vi "校准记录.vi"(8 "error in (no error)":errorcluster, 9 "曲线模型":T1={"标液浓度1"=0.0, "测量吸光度1"=0.0, "样品1启用"=FALSE, "标液浓度2"=0.0, "测量吸光度2"=0.0, "样品2启用"=FALSE, "标液浓度3"=0.0, "测量吸光度3"=0.0, "样品3启用"=FALSE, "标液浓度4"=0.0, "测量吸光度4"=0.0, "样品4启用"=FALSE, "标液浓度5"=0.0, "测量吸光度5"=0.0, "样品5启用"=FALSE, "模型"=enum."线性", "精度"=4.0, "XY图"=[], "拟合公式"="", "r^2"=0.0, "标样一校准时间"=timestamp(0 s since 1904-01-01), "标样二校准时间"=timestamp(0 s since 1904-01-01), "标样三校准时间"=timestamp(0 s since 1904-01-01), "标样四校准时间"=timestamp(0 s since 1904-01-01), "标样五校准时间"=timestamp(0 s since 1904-01-01), "二次方程"={"c"=0.0, "x"=0.0, "x^2"=0.0}, "标定时间"=timestamp(0 s since 1904-01-01), "拟合公式 2"="", "r^2 2"=0.0} {"r^2 2" format="%.7f"; "标定时间" format="%<%m/%d/%y %H:%M:%S>T"; "标样五校准时间" format="%<%m/%d/%y %H:%M:%S>T"; "标样四校准时间" format="%<%m/%d/%y %H:%M:%S>T"; "标样三校准时间" format="%<%m/%d/%y %H:%M:%S>T"; "标样二校准时间" format="%<%m/%d/%y %H:%M:%S>T"; "标样一校准时间" format="%<%m/%d/%y %H:%M:%S>T"; "r^2" format="%.7f"; "测量吸光度5" format="%#.6f"; "测量吸光度4" format="%#.6f"; "测量吸光度3" format="%#.6f"; "测量吸光度2" format="%#.6f"; "测量吸光度1" format="%#.6f"}, 10 "量程":enum16{"低量程", "高量程"}(ring), 11 "测量模式":string="所有测量模式") -> (0 "error out":errorcluster)   [LabVIEW 2016, in "斯坦道CODMn.lvlib"]
panel:
  out "结果字符串":string
  in  "data in":T2
  # "校准时间"
  # "标液浓度"
  # "吸光值显示"
  # "标液一"
  # "标液二"
  # "标液三"
  # "零点"
  # "跨度"
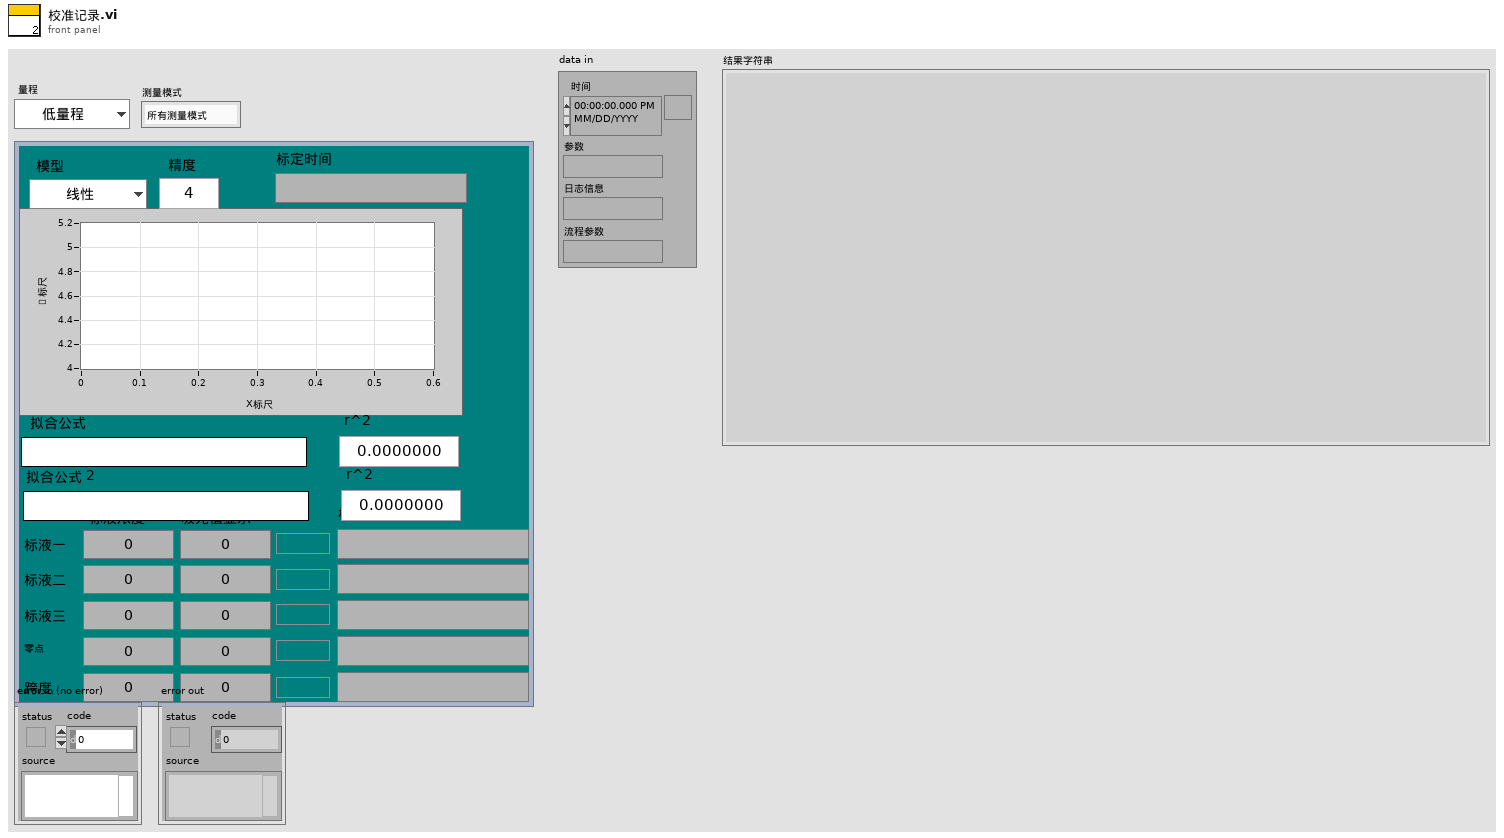
[diagram p1: front panel]
types:
  T1 = cluster{"标液浓度1":dbl, "测量吸光度1":dbl, "样品1启用":bool, "标液浓度2":dbl, "测量吸光度2":dbl, "样品2启用":bool, "标液浓度3":dbl, "测量吸光度3":dbl, "样品3启用":bool, "标液浓度4":dbl, "测量吸光度4":dbl, "样品4启用":bool, "标液浓度5":dbl, "测量吸光度5":dbl, "样品5启用":bool, "模型":enum32{"线性", "多项式", "折线"}, "精度":dbl, "XY图":cluster{"X Values":dbl[], "Y Values":dbl[]}[], "拟合公式":string, "r^2":dbl, "标样一校准时间":timestamp, "标样二校准时间":timestamp, "标样三校准时间":timestamp, "标样四校准时间":timestamp, "标样五校准时间":timestamp, "二次方程":cluster{"c":dbl, "x":dbl, "x^2":dbl}, "标定时间":timestamp, "拟合公式 2":string, "r^2 2":dbl}
  T2 = cluster{"时间":timestamp, "参数":string, "日志信息":string, "流程参数":string}
  T3 = cluster{"低标液1浓度":dbl, "低标液1信号值":dbl, "低标液1启用":u16, "低标液2浓度":dbl, "低标液2信号值":dbl, "低标液2启用":u16, "低标液3浓度":dbl, "低标液3信号值":dbl, "低标液3启用":u16, "低标液4浓度":dbl, "低标液4信号值":dbl, "低标液4启用":u16, "低标液5浓度":dbl, "低标液5信号值":dbl, "低标液5启用":u16, "高标液1浓度":dbl, "高标液1信号值":dbl, "高标液1启用":u16, "高标液2浓度":dbl, "高标液2信号值":dbl, "高标液2启用":u16, "高标液3浓度":dbl, "高标液3信号值":dbl, "高标液3启用":u16, "高标液4浓度":dbl, "高标液4信号值":dbl, "高标液4启用":u16, "高标液5浓度":dbl, "高标液5信号值":dbl, "高标液5启用":u16, "低斜率":dbl, "低截距":dbl, "低二次多项式系数":dbl, "低线性相关系数":dbl, "高斜率":dbl, "高截距":dbl, "高二次多项式系数":dbl, "高线性相关系数":dbl}
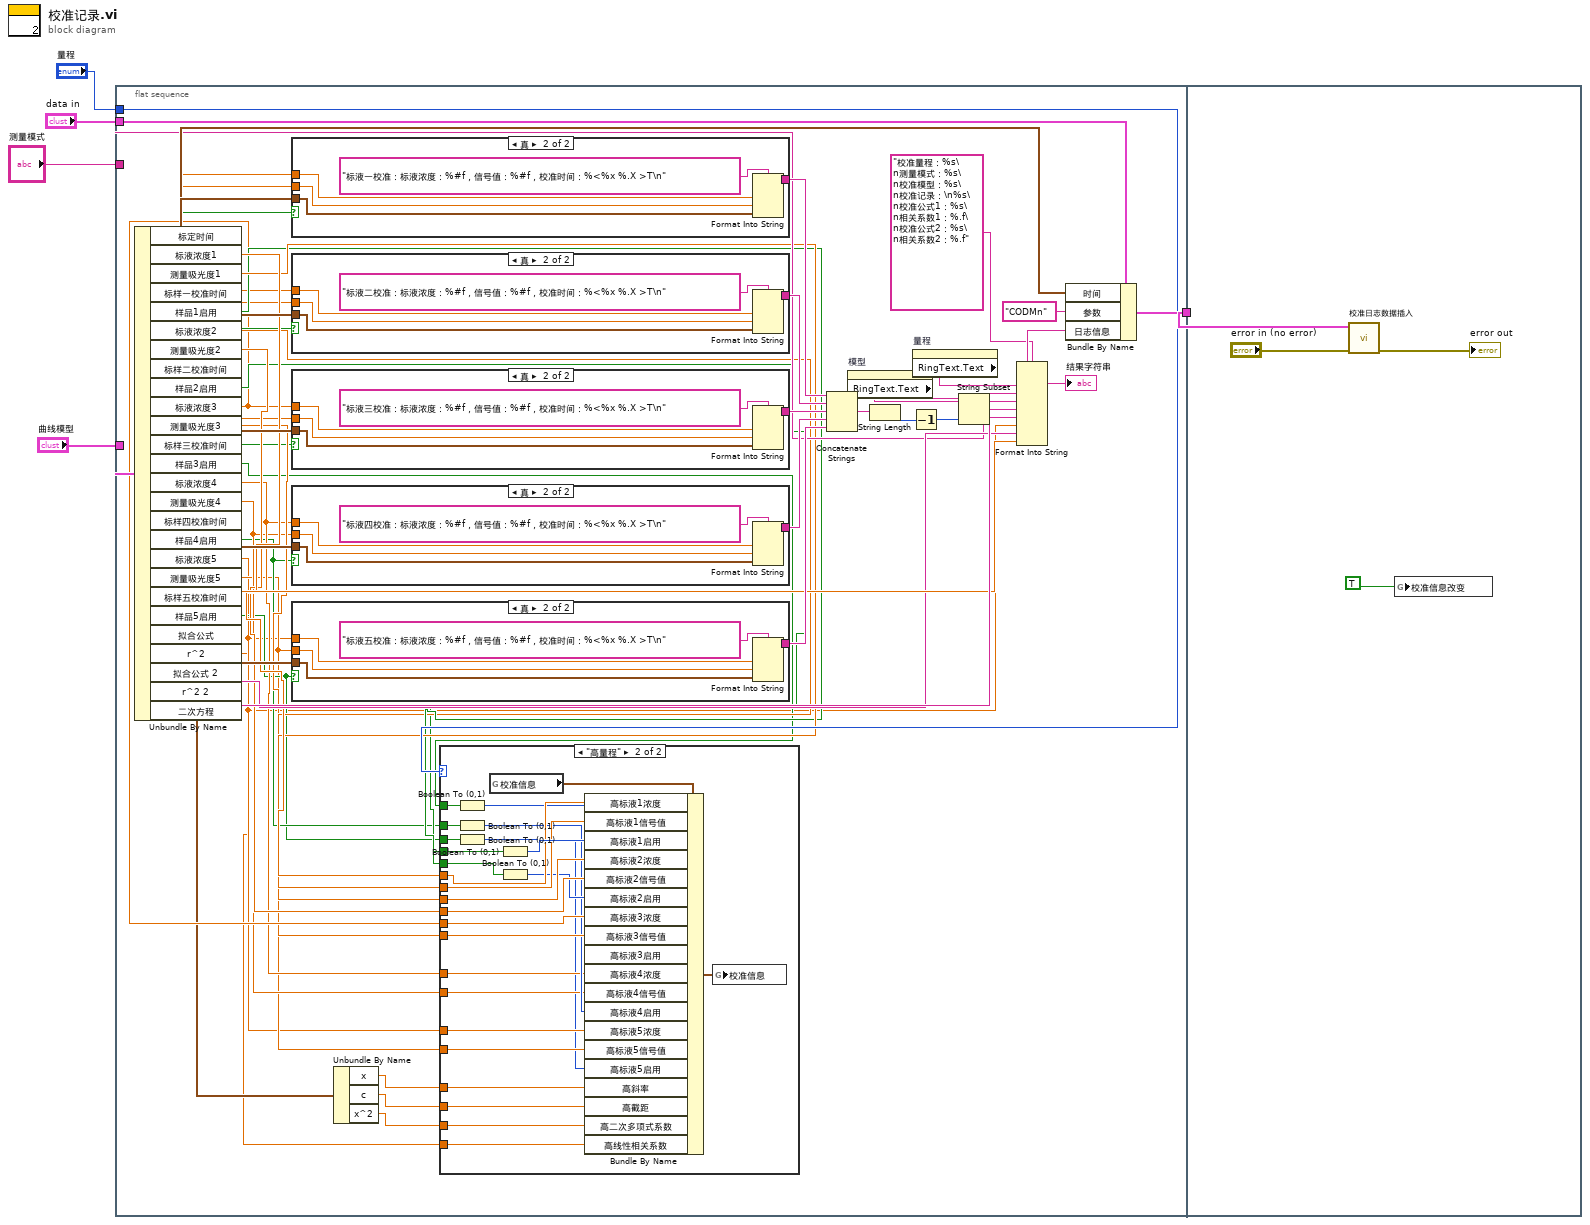
[diagram p0: block diagram]
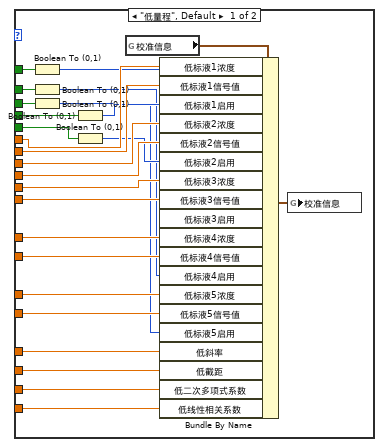
[diagram p2: hidden frame]
diagram:
  n1 = flat-sequence {
    tunnel: "量程" -> [w26]
    tunnel: "曲线模型" -> [w49]
    tunnel: "data in" -> [w53]
    tunnel: [w52] -> w2
    tunnel: "测量模式" -> [w27]
    tunnel: w2 -> [w132]
    frame #0 {
      n2 = Unbundle By Name(w49) -> ("标定时间"=w33:timestamp, "标液浓度1"=w25:dbl, "测量吸光度1"=w24:dbl, "标样一校准时间"=w48:timestamp, "样品1启用"=w23:bool, "标液浓度2"=w22:dbl, "测量吸光度2"=w21:dbl, "标样二校准时间"=w47:timestamp, "样品2启用"=w20:bool, "标液浓度3"=w19:dbl, "测量吸光度3"=w18:dbl, "标样三校准时间"=w46:timestamp, "样品3启用"=w17:bool, "标液浓度4"=w16:dbl, "测量吸光度4"=w15:dbl, "标样四校准时间"=w45:timestamp, "样品4启用"=w14:bool, "标液浓度5"=w11:dbl, "测量吸光度5"=w12:dbl, "标样五校准时间"=w44:timestamp, "样品5启用"=w13:bool, "拟合公式"=w38:string, "r^2"=w6:dbl, "拟合公式 2"=w31:string, "r^2 2"=w32:dbl, "二次方程"=w10:cluster{"c":dbl, "x":dbl, "x^2":dbl})
      n3 = case shown="真" w23 {
        tunnel: w25 -> [_ w129]
        tunnel: w24 -> [_ w128]
        tunnel: w48 -> [_ w127]
        tunnel: [_ w126] -> w43
        frame False {
        }
        frame True {
          n4 = Format Into String(format string="标液一校准：标液浓度：%#f，信号值：%#f，校准时间：%<%x %.X >T\n" ("格式字符串"), w129, w128, w127) -> (resulting string=w126:string)  [unwired: 2 in, 1 out]
        }
      }
      n5 = case shown="真" w20 {
        tunnel: w22 -> [_ w124]
        tunnel: w21 -> [_ w123]
        tunnel: w47 -> [_ w122]
        tunnel: [_ w121] -> w42
        frame False {
        }
        frame True {
          n6 = Format Into String(format string="标液二校准：标液浓度：%#f，信号值：%#f，校准时间：%<%x %.X >T\n" ("格式字符串"), w124, w123, w122) -> (resulting string=w121:string)  [unwired: 2 in, 1 out]
        }
      }
      n7 = case shown="真" w17 {
        tunnel: w19 -> [_ w119]
        tunnel: w18 -> [_ w118]
        tunnel: w46 -> [_ w117]
        tunnel: [_ w116] -> w41
        frame False {
        }
        frame True {
          n8 = Format Into String(format string="标液三校准：标液浓度：%#f，信号值：%#f，校准时间：%<%x %.X >T\n" ("格式字符串"), w119, w118, w117) -> (resulting string=w116:string)  [unwired: 2 in, 1 out]
        }
      }
      n9 = case shown="真" w14 {
        tunnel: w16 -> [_ w114]
        tunnel: w15 -> [_ w113]
        tunnel: w45 -> [_ w112]
        tunnel: [_ w111] -> w40
        frame False {
        }
        frame True {
          n10 = Format Into String(format string="标液四校准：标液浓度：%#f，信号值：%#f，校准时间：%<%x %.X >T\n" ("格式字符串"), w114, w113, w112) -> (resulting string=w111:string)  [unwired: 2 in, 1 out]
        }
      }
      n11 = case shown="真" w13 {
        tunnel: w11 -> [_ w109]
        tunnel: w12 -> [_ w108]
        tunnel: w44 -> [_ w107]
        tunnel: [_ w106] -> w39
        frame False {
        }
        frame True {
          n12 = Format Into String(format string="标液五校准：标液浓度：%#f，信号值：%#f，校准时间：%<%x %.X >T\n" ("格式字符串"), w109, w108, w107) -> (resulting string=w106:string)  [unwired: 2 in, 1 out]
        }
      }
      n13 = Unbundle By Name(w10) -> ("x"=w9:dbl, "c"=w8:dbl, "x^2"=w7:dbl)
      n14 = case shown="\"高量程\"" w26 {
        tunnel: w25 -> [w79 w103]
        tunnel: w24 -> [w78 w102]
        tunnel: w23 -> [w76 w105]
        tunnel: w22 -> [w77 w101]
        tunnel: w21 -> [w74 w100]
        tunnel: w20 -> [w73 w99]
        tunnel: w19 -> [w71 w97]
        tunnel: w18 -> [w70 w96]
        tunnel: w17 -> [w69 w95]
        tunnel: w16 -> [w67 w90]
        tunnel: w15 -> [w66 w91]
        tunnel: w14 -> [w65 w93]
        tunnel: w13 -> [w60 w89]
        tunnel: w12 -> [w62 w87]
        tunnel: w11 -> [w63 w88]
        tunnel: w9 -> [w57 w83]
        tunnel: w8 -> [w56 w82]
        tunnel: w7 -> [w55 w81]
        tunnel: w6 -> [w54 w80]
        frame "低量程", Default {
          n15 = Boolean To (0,1)(Boolean=w69) -> (0, 1=w68:i16)
          n16 = Boolean To (0,1)(Boolean=w65) -> (0, 1=w64:i16)
          n17 = Boolean To (0,1)(Boolean=w60) -> (0, 1=w61:i16)
          n18 = Boolean To (0,1)(Boolean=w76) -> (0, 1=w75:i16)
          n19 = Boolean To (0,1)(Boolean=w73) -> (0, 1=w72:i16)
          n20 = global read "CODMn断电保存全局变量.vi" "校准信息"() -> (w58:T3)
          n21 = Bundle By Name(cluster=w58, "低标液1浓度"=w79, "低标液1信号值"=w78, "低标液1启用"=w75, "低标液2浓度"=w77, "低标液2信号值"=w74, "低标液2启用"=w72, "低标液3浓度"=w71, "低标液3信号值"=w70, "低标液3启用"=w68, "低标液4浓度"=w67, "低标液4信号值"=w66, "低标液4启用"=w64, "低标液5浓度"=w63, "低标液5信号值"=w62, "低标液5启用"=w61, "低斜率"=w57, "低截距"=w56, "低二次多项式系数"=w55, "低线性相关系数"=w54) -> (w59:T3)
          n22 = global write "CODMn断电保存全局变量.vi" "校准信息"(w59) -> ()
        }
        frame "高量程" {
          n23 = Boolean To (0,1)(Boolean=w95) -> (0, 1=w94:i16)
          n24 = Boolean To (0,1)(Boolean=w93) -> (0, 1=w92:i16)
          n25 = Boolean To (0,1)(Boolean=w89) -> (0, 1=w86:i16)
          n26 = global read "CODMn断电保存全局变量.vi" "校准信息"() -> (w84:T3)
          n27 = Boolean To (0,1)(Boolean=w105) -> (0, 1=w104:i16)
          n28 = Boolean To (0,1)(Boolean=w99) -> (0, 1=w98:i16)
          n29 = Bundle By Name(cluster=w84, "高标液1浓度"=w103, "高标液1信号值"=w102, "高标液1启用"=w104, "高标液2浓度"=w101, "高标液2信号值"=w100, "高标液2启用"=w98, "高标液3浓度"=w97, "高标液3信号值"=w96, "高标液3启用"=w94, "高标液4浓度"=w90, "高标液4信号值"=w91, "高标液4启用"=w92, "高标液5浓度"=w88, "高标液5信号值"=w87, "高标液5启用"=w86, "高斜率"=w83, "高截距"=w82, "高二次多项式系数"=w81, "高线性相关系数"=w80) -> (w85:T3)
          n30 = global write "CODMn断电保存全局变量.vi" "校准信息"(w85) -> ()
        }
      }
      n31 = Concatenate Strings(w43, w42, w41, w40, w39) -> (w36:string)
      n32 = property on="模型" class="Enum (严格)"() -> ("RingText.Text"=w30:string)  [unwired: 2 in, 2 out]
      n33 = String Length(string=w36) -> (length=w35:i32)
      n34 = Decrement(x=w35) -> (x-1=w34:i32)
      n35 = property on="量程" class="Enum (严格)"() -> ("RingText.Text"=w28:string)  [unwired: 2 in, 2 out]
      n36 = String Subset(string=w36, length (rest)=w34) -> (substring=w37:string)  [unwired: 1 in]
      n37 = Format Into String(format string="校准量程：%s\n测量模式：%s\n校准模型：%s\n校准记录：\n%s\n校准公式1：%s\n相关系数1：%.f\n校准公式2：%s\n相关系数2：%.f" ("格式字符串"), w28, w27, w30, w37, w38, w6, w31, w32) -> (resulting string=w51:string)  [unwired: 2 in, 1 out]
      "结果字符串" <- w51
      n38 = Bundle By Name(cluster=w53, "时间"=w33, "参数"="CODMn", "日志信息"=w51) -> (w52:T2)
    }
    frame #1 {
      n39 = call "校准日志数据插入.vi"("data"=w132, "错误输入（无错误）"="error in (no error)") -> ("错误输出"=→"error out":errorcluster)  [unwired: 8 in]
      n40 = global write "CODMn断电保存全局变量.vi" "校准信息改变"(TRUE ("关键参数改变")) -> ()
    }
  }
